vi "SUB_USBDAQ_AudioLoopback.vi"(4 "AO Amplitude (V)":dbl=0.1, 5 "Frequency (Hz)":dbl=1000.0, 6 "input terminal configuration":i32(ring)=-1 items=["default"=-1, "RSE"=10083, "NRSE"=10078, "Differential"=10106, "Pseudodifferential"=12529], 7 "AI_Name_Receiving":string, 8 "AO_Name_Sending":string) -> (0 "THD%":dbl format="%.4f", 1 "THD+N(%)":dbl format="%.2f", 2 "rms value":dbl format="%0.2f", 3 "detected fundamental\nfrequency [Hz]":dbl format="%.6f")   [LabVIEW 2011]
uses:
  <vilib>/DAQmx/write.llb/DAQmx Write (Analog 1D DBL 1Chan NSamp).vi
  <vilib>/DAQmx/configure/timing.llb/DAQmx Timing (Sample Clock).vi
  <vilib>/DAQmx/read.llb/DAQmx Read (Analog 1D DBL 1Chan NSamp).vi
  <vilib>/Analysis/NI_AALBase.lvlib
  <vilib>/DAQmx/create/channels.llb/DAQmx Create Channel (AI-Voltage-Basic).vi
  <vilib>/addons/Sound and Vibration/svt_Subset FFT/SVT Power Spectrum Subset (1 Ch).vi
  <vilib>/addons/Sound and Vibration/svt_Distortion/SVT THD+N (Time) (1 Ch).vi
  <vilib>/DAQmx/create/channels.llb/DAQmx Create Channel (AO-Voltage-Basic).vi
  <vilib>/addons/Sound and Vibration/svt_Distortion/SVT THD and Harmonic Components (Time) (1 Ch).vi
  C:/Program Files (x86)/National Instruments/LabVIEW 2011/resource/objmgr/daqmx.rc
  <vilib>/Analysis/NI_AALPro.lvlib
  <vilib>/Analysis/5stat.llb/RMS (DBL).vi
panel:
  out "detected fundamental\namplitude 2":dbl format="%.2f"
  out "Waveform Chart":dbl[](graph)
  out "detected fundamental\namplitude":dbl format="%.6f"
  in  "frequency range":T1={"start frequency"=100.0, "stop frequency"=10000.0} {"stop frequency" min=0.0 format="%.2f"; "start frequency" min=0.0 format="%.2f"}
  out "Waveform Graph":cluster{"f0":dbl, "df":dbl, "magnitude":dbl[]}(graph)
  out "error out":errorcluster
  out "task out":refnum<k21>
  in  "error in":errorcluster
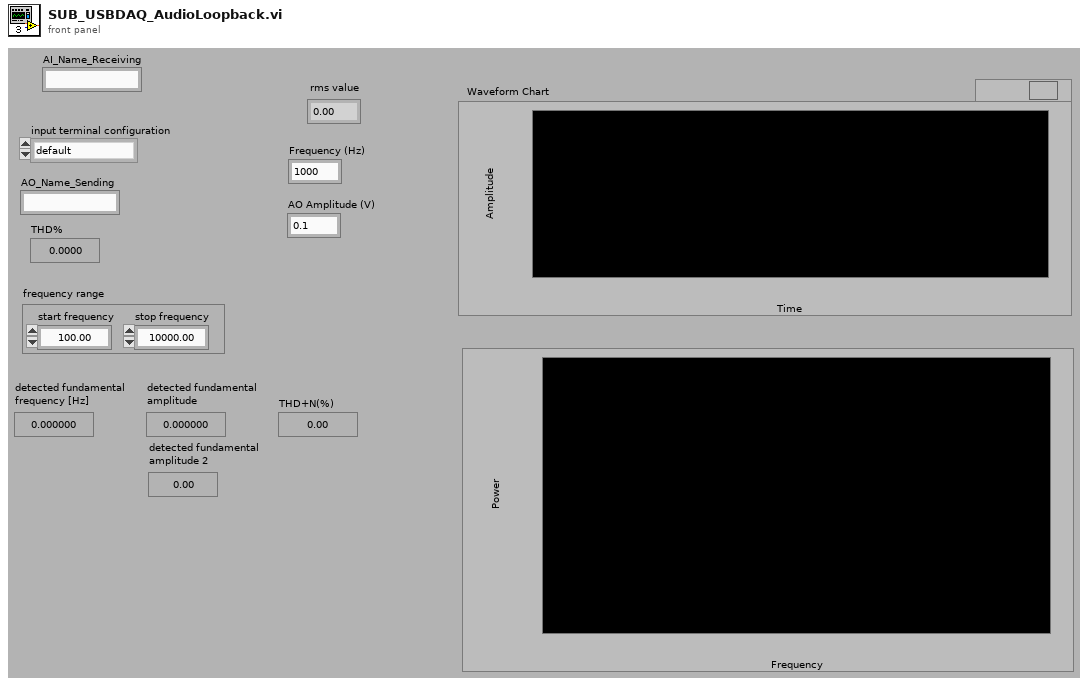
[diagram p1: front panel]
types:
  T1 = cluster{"start frequency":dbl, "stop frequency":dbl}
  T2 = cluster{"THD units":enum16{"dB", "linear ratio", "%"}, "harmonic component amplitude units":enum16{"EU rms", "EU peak", "EU peak-peak", "dB ref fund"}, "detected fundamental amplitude units":enum16{"EU rms", "EU peak", "EU peak-peak"}}
  T3 = cluster{"THD+N units":enum16{"dB", "linear ratio", "%"}, "detected fundamental amplitude units":enum16{"EU rms", "EU peak", "EU peak-peak"}}
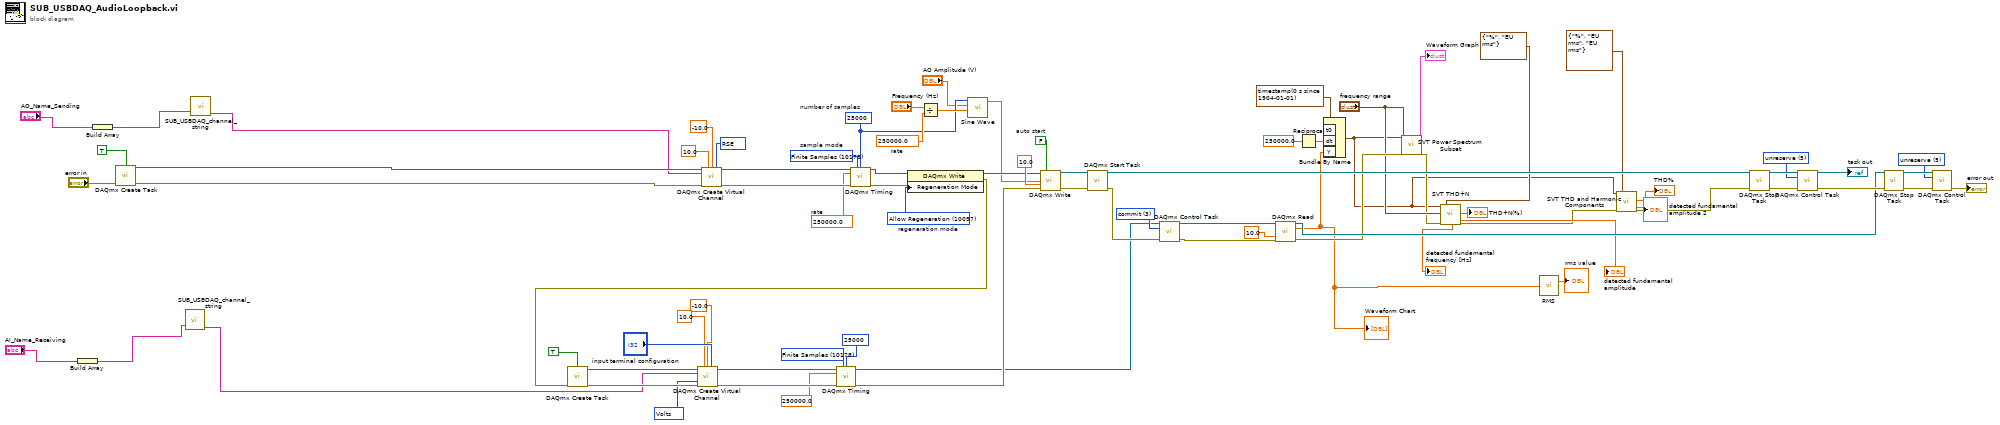
[diagram p0: block diagram]
diagram:
  w20 = 10083 items=["Default"=-1, "RSE"=10083, "Differential"=10106, "Pseudodifferential"=12529] ("output terminal configuration")
  w31 = 10348 items=["Volts"=10348, "From Custom Scale"=10065] ("units")
  w39 = 5 items=["verify"=2, "reserve"=4, "commit"=3, "unreserve"=5, "abort"=6] ("action")
  w43 = 250000.0  # rate
  w53 = 5 items=["verify"=2, "reserve"=4, "commit"=3, "unreserve"=5, "abort"=6] ("action")
  w57 = 3 items=["verify"=2, "reserve"=4, "commit"=3, "unreserve"=5, "abort"=6] ("action")
  w59 = 10178 items=["Finite Samples"=10178, "Continuous Samples"=10123, "Hardware Timed Single Point"=12522] ("sample mode")
  w71 = FALSE  # auto start
  w72 = 10097 items=["Allow Regeneration"=10097, "Do Not Allow Regeneration"=10158]  # regeneration mode
  w73 = 10178 items=["Finite Samples"=10178, "Continuous Samples"=10123, "Hardware Timed Single Point"=12522]  # sample mode
  w74 = 250000.0  # rate
  w37 = 25000  # number of samples
  n1 = Build Array("AI_Name_Receiving") -> (w4:string[])
  n2 = Build Array("AO_Name_Sending") -> (w5:string[])
  n3 = call <vilib>:"DAQmx Create Task.vi"("auto cleanup"=TRUE, "error in"="error in") -> ("task out"=w81:refnum<k21>, "error out"=w80:errorcluster)  [unwired: 12 in]
  n4 = call "SUB_USBDAQ_channel_string.vi"("channel"=w4) -> ("resulting string"=w3:string)  [unwired: 1 in, 2 out]
  n5 = call "SUB_USBDAQ_channel_string.vi"("channel"=w5) -> ("resulting string"=w6:string)  [unwired: 1 in, 2 out]
  n6 = call-poly <vilib>:"DAQmx Create Virtual Channel.vi"("task in"=w81, "maximum value"=10.0, "minimum value"=-10.0, "output terminal configuration"=w20, "physical channels"=w6, "error in"=w80) -> ("task out"=w78:refnum<k21>, "error out"=w77:errorcluster)  [unwired: 8 in]
  n7 = call-poly <vilib>:"DAQmx Timing.vi"("task/channels in"=w78, "sample mode"=w73, "samples per channel"=w37, "rate"=w74, "error in"=w77) -> ("task out"=w76:refnum<k21>, "error out"=w75:errorcluster)  [unwired: 9 in]
  n8 = property class="DAQmx Write"(reference=w76, error in=w75, "Regeneration Mode"=w72) -> (reference out=w65:refnum<k21>, error out=w50:errorcluster)
  n9 = call <vilib>:"DAQmx Create Task.vi"("auto cleanup"=TRUE, "error in"=w50) -> ("task out"=w63:refnum<k21>, "error out"=w62:errorcluster)  [unwired: 12 in]
  n10 = call-poly <vilib>:"DAQmx Create Virtual Channel.vi"("task in"=w63, "maximum value"=10.0, "minimum value"=-10.0, "input terminal configuration"="input terminal configuration", "physical channels"=w3, "units"=w31, "error in"=w62) -> ("task out"=w52:refnum<k21>, "error out"=w61:errorcluster)  [unwired: 7 in]
  n11 = call-poly <vilib>:"DAQmx Timing.vi"("task/channels in"=w52, "sample mode"=w59, "samples per channel"=25000, "rate"=250000.0, "error in"=w61) -> ("task out"=w47:refnum<k21>, "error out"=w49:errorcluster)  [unwired: 9 in]
  n12 = Divide(x="Frequency (Hz)", y=w43) -> (x/y=w44:dbl)
  n13 = call <vilib>:"Sine Wave.vi"("samples"=w37, "amplitude"="AO Amplitude (V)", "frequency"=w44) -> ("sine wave"=w35:dbl[])  [unwired: 2 in, 2 out]
  n14 = call-poly <vilib>:"DAQmx Write.vi"("task/channels in"=w65, "auto start"=w71, "data"=w35, "timeout"=10.0 ("timeout (s)"), "error in"=w49) -> ("task out"=w70:refnum<k21>, "error out"=w69:errorcluster)  [unwired: 8 in, 1 out]
  n15 = call <vilib>:"DAQmx Start Task.vi"("task/channels in"=w70, "error in"=w69) -> ("task out"=w67:refnum<k21>, "error out"=w48:errorcluster)  [unwired: 12 in]
  n16 = call <vilib>:"DAQmx Control Task.vi"("task/channels in"=w47, "action"=w57, "error in"=w48) -> ("task out"=w23:refnum<k21>, "error out"=w22:errorcluster)  [unwired: 11 in]
  n17 = call-poly <vilib>:"DAQmx Read.vi"("task/channels in"=w23, "timeout"=10.0, "error in"=w22) -> ("task out"=w45:refnum<k21>, "data"=w8:dbl[], "error out"=w30:errorcluster)  [unwired: 10 in]
  "Waveform Chart" <- w8
  n18 = Reciprocal(x=250000.0) -> (1/x=w34:dbl)
  n19 = Bundle By Name("t0"=timestamp(0 s since 1904-01-01), "dt"=w34, "Y"=w8) -> (w9:waveform(dbl))  [unwired: 1 in]
  n20 = call-poly <vilib>:"SVT Power Spectrum Subset.vi"("scaled signal [EU]"=w9, "frequency range"="frequency range", "error in (no error)"=w30) -> ("power spectrum [dB EU]"=→"Waveform Graph":cluster{"f0":dbl, "df":dbl, "magnitude":dbl[]}, "error out"=w27:errorcluster)  [unwired: 11 in, 4 out]
  n21 = call-poly <vilib>:"SVT THD+N.vi"("scaled signal [EU]"=w9, "frequency range"="frequency range", "error in (no error)"=w27, "desired units"=T3 {"THD+N units"=enum."%", "detected fundamental amplitude units"=enum."EU rms"}) -> ("detected fundamental\nfrequency [Hz]"=→"detected fundamental\nfrequency [Hz]":dbl, "detected fundamental\namplitude"=→"detected fundamental\namplitude":dbl, "THD+N"=→"THD+N(%)":dbl, "error out"=w14:errorcluster)  [unwired: 10 in, 2 out]
  n22 = call-poly <vilib>:"RMS.vi"("X"=w8) -> ("rms value"=→"rms value":dbl)  [unwired: 1 out]
  n23 = call-poly <vilib>:"SVT THD and Harmonic Components.vi"("scaled signal [EU]"=w9, "error in (no error)"=w14, "desired units"=T2 {"THD units"=enum."%", "harmonic component amplitude units"=enum."EU rms", "detected fundamental amplitude units"=enum."EU rms"}) -> ("detected fundamental\namplitude"=→"detected fundamental\namplitude 2":dbl, "THD"=→"THD%":dbl, "error out"=w15:errorcluster)  [unwired: 9 in, 5 out]
  n24 = call <vilib>:"DAQmx Stop Task.vi"("task/channels in"=w67, "error in"=w15) -> ("task out"=w40:refnum<k21>, "error out"=w41:errorcluster)  [unwired: 12 in]
  n25 = call <vilib>:"DAQmx Control Task.vi"("task/channels in"=w40, "action"=w39, "error in"=w41) -> ("task out"=→"task out":refnum<k21>, "error out"=w46:errorcluster)  [unwired: 11 in]
  n26 = call <vilib>:"DAQmx Stop Task.vi"("task/channels in"=w45, "error in"=w46) -> ("task out"=w55:refnum<k21>, "error out"=w54:errorcluster)  [unwired: 12 in]
  n27 = call <vilib>:"DAQmx Control Task.vi"("task/channels in"=w55, "action"=w53, "error in"=w54) -> ("error out"=→"error out":errorcluster)  [unwired: 11 in, 1 out]
